vi "Read IMU Gyro.vi"(0 "I2CDevRef":T1={"DevStatus"={"status"=FALSE, "code"=0, "source"=""}, "Controller"=enum."Controller 1", "Device Address"=0, "Handle"=0, "I2C Bus"=enum."Invalid"} {"Device Address" format="%.0x"}) -> (3 "I2CDevRef 2":T1={"DevStatus"={"status"=FALSE, "code"=0, "source"=""}, "Controller"=enum."Controller 1", "Device Address"=0, "Handle"=0, "I2C Bus"=enum."Invalid"} {"Device Address" format="%.0x"}, 4 "X":dbl, 6 "Y":dbl, 8 "Z":dbl, 12 "Raw X":dbl, 13 "Raw Y":dbl, 14 "Raw Z":dbl)   [LabVIEW 2014]
uses:
  <vilib>/Rock Robotics/WPI/I2C/WPI_I2CDevRef.ctl
  <vilib>/Rock Robotics/SystemInterfaces/Typedef/FPGA_TypedefDigitalModule.ctl
  <vilib>/Rock Robotics/SystemInterfaces/i2clib/i2c_bus.ctl
  Robot Global Data.vi
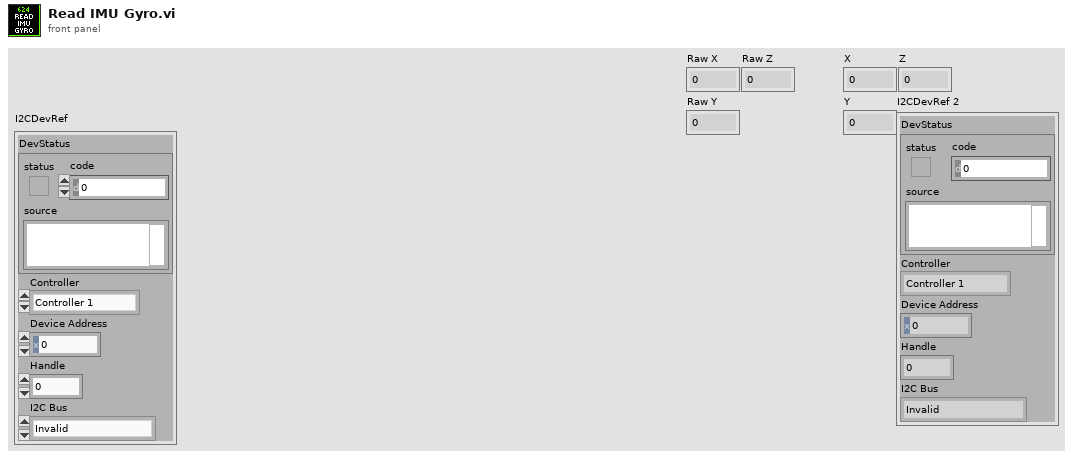
[diagram p1: front panel]
types:
  T1 = typedef "WPI_I2CDevRef.ctl" = cluster{"DevStatus":errorcluster, "Controller":T2, "Device Address":u8, "Handle":i32, "I2C Bus":T3}
  T2 = typedef "FPGA_TypedefDigitalModule.ctl" = enum16{"Controller 1"}
  T3 = typedef "i2c_bus.ctl" = enum16{"I2C On-Board", "I2C MXP", "Invalid"}
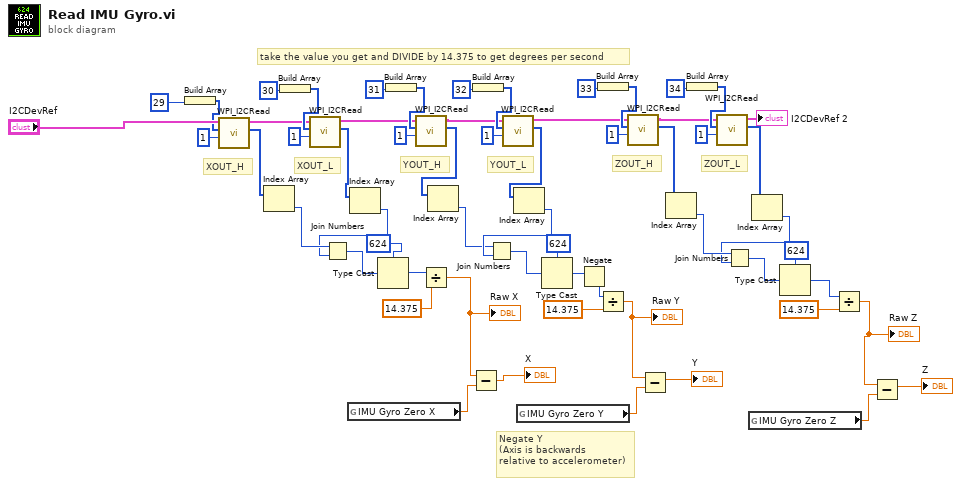
[diagram p0: block diagram]
diagram:
  # "Negate Y\n(Axis is backwards\nrelative to accelerometer)"
  # "take the value you get and DIVIDE by 14.375 to get degrees per second"
  # "ZOUT_L"
  # "ZOUT_H"
  # "YOUT_L"
  # "YOUT_H"
  # "XOUT_L"
  # "XOUT_H"
  n1 = Build Array(u8 29) -> (w57:u8[])
  n2 = call <vilib>:"WPI_I2CRead.vi"("I2CBytesToRead"=u8 1, "I2CRegister"=w57, "I2CDevRef"="I2CDevRef") -> ("Data Out"=w35:u8[], "I2CDevRef"=w52:T1)  [unwired: 6 in, 1 out]
  n3 = Index Array(array=w35) -> (element=w33:u8)  [unwired: 1 in]
  n4 = Build Array(u8 30) -> (w54:u8[])
  n5 = call <vilib>:"WPI_I2CRead.vi"("I2CBytesToRead"=u8 1, "I2CRegister"=w54, "I2CDevRef"=w52) -> ("Data Out"=w34:u8[], "I2CDevRef"=w48:T1)  [unwired: 6 in, 1 out]
  n6 = global read "Robot Global Data.vi" "IMU Gyro Zero X"() -> (w5:dbl)
  n7 = Index Array(array=w34) -> (element=w32:u8)  [unwired: 1 in]
  n8 = Join Numbers(hi=w33, lo=w32) -> ((hi.lo)=w31:u16)
  n9 = Type Cast(type=i16 624, x=w31) -> (*(type *) &x=w17:i16)
  n10 = Build Array(u8 31) -> (w50:u8[])
  n11 = call <vilib>:"WPI_I2CRead.vi"("I2CBytesToRead"=u8 1, "I2CRegister"=w50, "I2CDevRef"=w48) -> ("Data Out"=w19:u8[], "I2CDevRef"=w44:T1)  [unwired: 6 in, 1 out]
  n12 = Divide(x=w17, y=14.375) -> (x/y=w4:dbl)
  "Raw X" <- w4
  n13 = Index Array(array=w19) -> (element=w26:u8)  [unwired: 1 in]
  n14 = Subtract(x=w4, y=w5) -> (x-y=→"X":dbl)
  n15 = Build Array(u8 32) -> (w46:u8[])
  n16 = call <vilib>:"WPI_I2CRead.vi"("I2CBytesToRead"=u8 1, "I2CRegister"=w46, "I2CDevRef"=w44) -> ("Data Out"=w18:u8[], "I2CDevRef"=w36:T1)  [unwired: 6 in, 1 out]
  n17 = Index Array(array=w18) -> (element=w27:u8)  [unwired: 1 in]
  n18 = Join Numbers(hi=w26, lo=w27) -> ((hi.lo)=w28:u16)
  n19 = global read "Robot Global Data.vi" "IMU Gyro Zero Y"() -> (w8:dbl)
  n20 = Type Cast(type=i16 624, x=w28) -> (*(type *) &x=w2:i16)
  n21 = Negate(x=w2) -> (-x=w1:i16)
  n22 = Build Array(u8 33) -> (w42:u8[])
  n23 = Divide(x=w1, y=14.375) -> (x/y=w7:dbl)
  "Raw Y" <- w7
  n24 = call <vilib>:"WPI_I2CRead.vi"("I2CBytesToRead"=u8 1, "I2CRegister"=w42, "I2CDevRef"=w36) -> ("Data Out"=w21:u8[], "I2CDevRef"=w37:T1)  [unwired: 6 in, 1 out]
  n25 = Subtract(x=w7, y=w8) -> (x-y=→"Y":dbl)
  n26 = Index Array(array=w21) -> (element=w25:u8)  [unwired: 1 in]
  n27 = Build Array(u8 34) -> (w39:u8[])
  n28 = call <vilib>:"WPI_I2CRead.vi"("I2CBytesToRead"=u8 1, "I2CRegister"=w39, "I2CDevRef"=w37) -> ("Data Out"=w20:u8[], "I2CDevRef"=→"I2CDevRef 2":T1)  [unwired: 6 in, 1 out]
  n29 = global read "Robot Global Data.vi" "IMU Gyro Zero Z"() -> (w10:dbl)
  n30 = Index Array(array=w20) -> (element=w24:u8)  [unwired: 1 in]
  n31 = Join Numbers(hi=w25, lo=w24) -> ((hi.lo)=w23:u16)
  n32 = Type Cast(type=i16 624, x=w23) -> (*(type *) &x=w13:i16)
  n33 = Divide(x=w13, y=14.375) -> (x/y=w11:dbl)
  "Raw Z" <- w11
  n34 = Subtract(x=w11, y=w10) -> (x-y=→"Z":dbl)
